vi "Main.vi"() -> ()   [LabVIEW 2020, in "Array Example.lvlib"]
uses:
  Array Example.lvlib
  OOPanel/ArrayManager/ArrayManager.lvclass
  Element B/Element B.lvclass
  Element Base/Element Base.lvclass
  Element A/Element A.lvclass
  <vilib>/platform/TimedLoop/XDataNode/XDataNode.xnode
  <vilib>/Platform/TimedLoop/XDataNode/nitl_modes.ctl
  <vilib>/Platform/TimedLoop/XDataNode/XDNodeRunTimeDep.lvlib
  <vilib>/Platform/TimedLoop/XDataNode/wakeup.ctl
  <vilib>/Platform/TimedLoop/XDataNode/timing_clust.ctl
panel:
  out "Stop":bool
  out "Values":string[](array[string])
  # "Note: If left to the default 1000 panel instances, this VI is expected to take a bit to start."
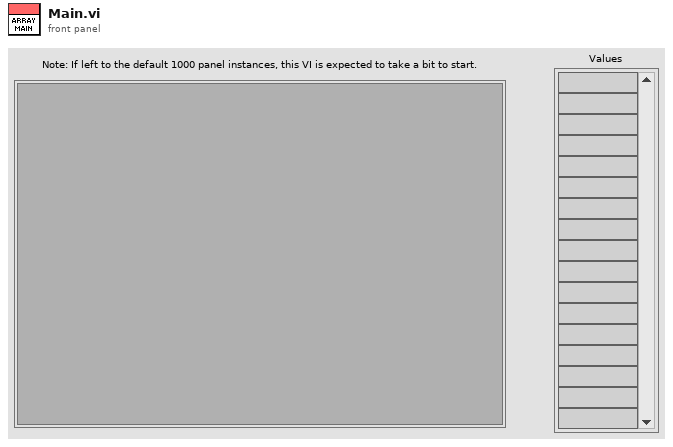
[diagram p1: front panel]
types:
  T1 = typedef "XDNodeRunTimeDep.lvlib/timing_clust.ctl" = cluster{"Expected End [f-1]":u64, "Actual End [f-1]":u64, "Finished Late? [f-1]":bool, "Expected End [i-1]":u64, "Actual End [i-1]":u64, "Finished Late? [i-1]":bool, "Expected Start [i]":u64, "Actual Start [i]":u64, "Expected Start [f]":u64, "Actual Start [f]":u64, "Source Name":string, "Structure Name":string, "Period":i64, "Deadline":i64, "Offset":i64, "Start":i64, "Priority":i32, "Timeout":i32, "Mode":T2, "Wakeup Reason":T3, "Error":errorcluster, "Source Type":string, "Secondary Source Type":string, "Global End Time":u64, "Global Start Time":u64, "Frame Duration":u64, "Iteration Duration":u64, "Assigned CPU":i32, "I/O Scan Engine Mode":u32}
  T2 = typedef "XDNodeRunTimeDep.lvlib/nitl_modes.ctl" = enum32{"No Change", "Process missed periods, maintain original phase", "Discard missed periods, maintain original phase", "Process missed periods, ignore original phase", "Discard missed periods, ignore original phase"}
  T3 = typedef "XDNodeRunTimeDep.lvlib/wakeup.ctl" = enum32{"Normal", "Aborted", "Asynchronous wakeup", "Timing source error", "Timed loop error", "Timeout"}
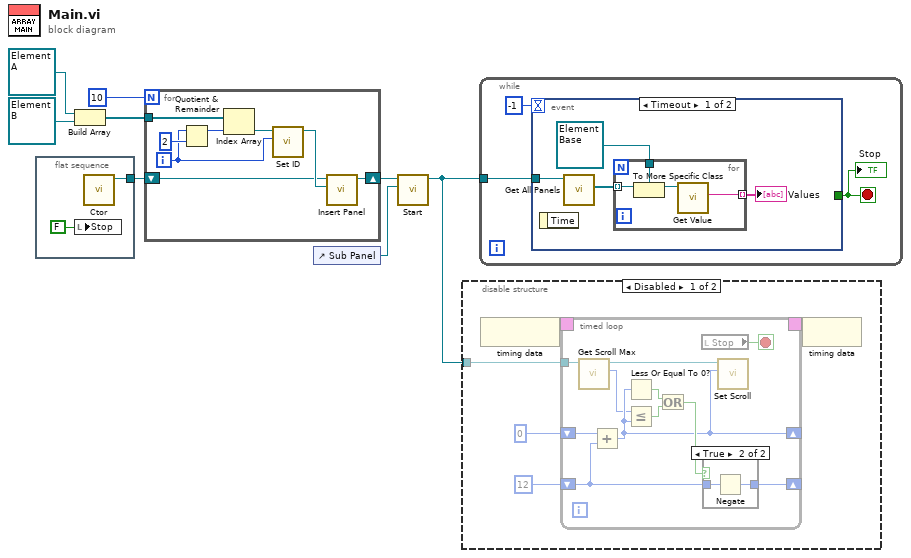
[diagram p0: block diagram]
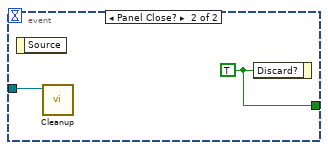
[diagram p4: hidden frame]
diagram:
  n1 = flat-sequence {
    tunnel: [w10] -> w8
    frame #0 {
      n2 = local write "Stop"(FALSE ("Stop")) -> ()
      n3 = call "Ctor.vi"() -> ("PanelArray"=w10:refnum<class "ArrayManager.lvclass">)  [unwired: 10 in, 1 out]
    }
  }
  n4 = Build Array(refnum<class "Element A.lvclass"> refnum ("Array Example.lvlib:Element A.lvclass"), refnum<class "Element B.lvclass"> refnum ("Array Example.lvlib:Element B.lvclass")) -> (w6:refnum<class "Element Base.lvclass">[])
  n5 = for {
    N: 10 -> [_]
    tunnel: w6 -> [w17]
    shift-right: [w14] -> w4
    shift-left: w8 -> [w11]
    i -> [w15]
    n6 = Quotient & Remainder(x=w15, y=2) -> (x-y*floor(x/y)=w16:i32)  [unwired: 1 out]
    n7 = Index Array(array=w17, index=w16) -> (element=w13:refnum<class "Element Base.lvclass">)
    n8 = call "Set ID.vi"("ID"=w15, "Element Base in"=w13) -> ("Element Base out"=w12:refnum<class "Element Base.lvclass">)  [unwired: 8 in, 1 out]
    n9 = call "Insert Panel.vi"("Panel/Type"=w12, "PanelArray in"=w11) -> ("PanelArray out"=w14:refnum<class "ArrayManager.lvclass">)  [unwired: 7 in, 2 out]
  }
  n10 = control-ref of="Sub Panel"() -> (w3:refnum<vi>)
  n11 = call "Start.vi"("Container"=w3, "ArrayManager in"=w4) -> ("ArrayManager out"=w1:refnum<class "ArrayManager.lvclass">)  [unwired: 8 in, 1 out]
  n12 = disable-structure shown="Disabled" {
    disable-tunnel: w1 -> [w19 _]
    frame Disabled {
      n13 = node-c288() -> (w23:T1)
      n14 = timed-loop {
        timing: w23 -> [_]
        timing-out: [_] -> w22
        tunnel: w19 -> [w25]
        shift-right: [w28] -> _
        shift-left: 0 -> [w34]
        shift-right: [w29] -> _
        shift-left: 12 -> [w30]
        stop <- w24 stop-if-true
        n15 = call "Get Scroll Max.vi"("ArrayManager in"=w25) -> ("Scroll Max"=w27:i32, "ArrayManager out"=w26:refnum<class "ArrayManager.lvclass">)  [unwired: 8 in, 1 out]
        n16 = Add(x=w34, y=w30) -> (x+y=w28:i32)
        n17 = Less Or Equal To 0?(x=w28) -> (x <= 0?=w33:bool)
        n18 = Less Or Equal?(x=w27, y=w28) -> (x <= y?=w32:bool)
        n19 = Or(x=w33, y=w32) -> (x .or. y?=w31:bool)
        n20 = local read "Stop"() -> (w24:bool)
        n21 = case shown="True" w31 {
          tunnel: w30 -> [w35 w37]
          tunnel: [w35 w36] -> w29
          frame False {
          }
          frame True {
            n22 = Negate(x=w37) -> (-x=w36:i32)
          }
        }
        n23 = call "Set Scroll.vi"("Position"=w28, "ArrayManager in"=w26) -> ()  [unwired: 8 in, 2 out]
      }
      n24 = node-c288(w22) -> ()
    }
    frame Enabled {
    }
  }
  n25 = while {
    tunnel: w1 -> [w43]
    stop <- w42 stop-if-true
    n26 = event shown="[0] Timeout" {
      selector: _ -> [_ _]
      dyn-events: _ -> [_ _]
      timeout: -1 -> [_ _]
      tunnel: w43 -> [w48 w53]
      tunnel: [_ w54] -> w42
      event Timeout {
        n27 = event-data() -> ()  [unwired: 1 in, 1 out]
        n28 = call "Get All Panels.vi"("PanelArray in"=w48) -> ("Panels"=w47:refnum<class "ArrayPanel.lvclass">[])  [unwired: 8 in, 2 out]
        n29 = for {
          tunnel: w47 -> [w52] mode=indexing
          tunnel: refnum<class "Element Base.lvclass"> refnum ("Array Example.lvlib:Element Base.lvclass") -> [w51]
          tunnel: [w49] -> w45 mode=indexing
          n30 = To More Specific Class(target class=w51, reference=w52) -> (specific class reference=w50:refnum<class "Element Base.lvclass">)  [unwired: 1 in, 1 out]
          n31 = call-dynamic "Get Value.vi"("Element Base in"=w50) -> ("Value"=w49:string)  [unwired: 8 in, 2 out]
        }
        "Values" <- w45
      }
      event Panel Close? {
        w54 = TRUE ("Discard?")
        n32 = event-data() -> ()  [unwired: 1 in, 1 out]
        n33 = call "Cleanup.vi"("PanelArray in"=w53) -> ()  [unwired: 10 in, 1 out]
        n34 = event-data("Discard?"=w54) -> ()  [unwired: 1 in, 1 out]
      }
    }
    "Stop" <- w42
  }
